vi "logical_series.resolve_batch.vi"(8 "error in":errorcluster, 10 "Data":T1, 11 "Nominal Client in":refnum<class "Nominal Client.lvclass">) -> (0 "error out":errorcluster, 1 "Response Headers":refnum<class "Response Headers.lvclass">, 2 "Response":string, 3 "Nominal Client out":refnum<class "Nominal Client.lvclass">)   [LabVIEW 2020, in "Nominal Client.lvclass"]
doc: "Resolves groups of channels, datasources and tags into logical series rids. An error response is provided if the channel + datasource + tag cannot be resolved into a logical series rid."
uses:
  Nominal Client.lvclass
  <vilib>/addons/_JKI.lib/REST Client/classes/Response Headers/Response Headers.lvclass
  d51cee68-3910-4483-a6bc-435354615454.vi
  <vilib>/JDP Science/JSONtext/Variant to JSON Text.vi
  <vilib>/JDP Science/JSONtext/LVClass Serializer/JSONtext LVClass Serializer.lvclass
  Nominal Client.lvclass/Nominal Client.ctl
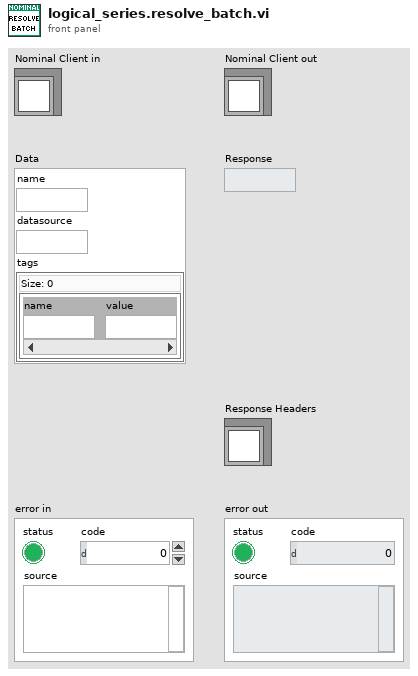
[diagram p1: front panel]
types:
  T1 = cluster{"name":string, "datasource":string, "tags":map{string, string}}
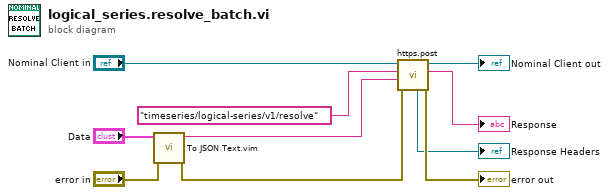
[diagram p0: block diagram]
diagram:
  n1 = call "To JSON Text.vim"("error in (no error)"="error in", "Anything"="Data") -> ("error out"=w1:errorcluster, "<JSON>"=w3:string)  [unwired: 8 in]
  n2 = call "https.post.vi"("error in"=w1, "Request body"=w3, "Path"="timeseries/logical-series/v1/resolve", "Nominal Client in"="Nominal Client in") -> ("error out"=→"error out":errorcluster, "Response"=→"Response":string, "Nominal Client out"=→"Nominal Client out":refnum<class "Nominal Client.lvclass">, "Response Headers"=→"Response Headers":refnum<class "Response Headers.lvclass">)  [unwired: 4 in]
